vi "Tank1 GO!.vi"() -> ()   [LabVIEW 2012]
doc: "This VI demonstrates how to control a simulated Robotics Starter Kit 2.0 robot. With a few modifications, you can deploy this VI to the Single-Board RIO 9632 on a real robot, and it runs on the real-time controller. For more information about how to modify this VI so you can deploy it to real hardware, refer to the <B>Robotics Module>>Simulating Mobile Robots</B> book on the <B>Contents</B> tab of the LabVIEW Help."
uses:
  <vilib>/Platform/TimedLoop/XDataNode/timing_clust.ctl
  <vilib>/Platform/TimedLoop/XDataNode/nitl_modes.ctl
  <vilib>/Platform/TimedLoop/XDataNode/wakeup.ctl
  <vilib>/robotics/Starter Kit/2.0/9632 Host Interface/NI_Robotics_Starter Kit Host_9632_2.0.lvclass
  <vilib>/Utility/AngleManip/Degrees to Radians (Scalar DBL).vi
  <vilib>/FPGAPlugInAG/sbRIO-9632/niLvFpga_Open_sbRIO-9632.vi
  <vilib>/rvi/interface/common/dynamic/niFpgaDynamicAddResources.vi
  <vilib>/robotics/Steering/Steering Frame/Apply Steering Frame Velocity to Motors.vi
  <vilib>/FPGAPlugInAG/Dynamic/niLvFpga_Close_Dynamic.vi
  <vilib>/Platform/TimedLoop/XDataNode/XDataNode.xnode
  <vilib>/rvi/interface/nirviOpenFPGA/nirviOpenFPGA.xnode
  FPGA Bitfiles/mainframe_FPGATarget_FPGA-conrolofTan_P2Uk2TjUNj0.lvbitx
  <vilib>/rvi/interface/nirviCloseFPGA/nirviCloseFPGA.xnode
  <vilib>/Platform/TimedLoop/XDataNode/XDNodeRunTimeDep.lvlib
  <vilib>/Utility/AngleManip/NI_AngleManipulation.lvlib
  <vilib>/robotics/Utilities/Scan Angles/NI_Robotics_Scan Angles.lvlib
  <vilib>/robotics/Steering/Steering Frame/NI_Robotics_Steering Frame.lvclass
  <vilib>/robotics/Starter Kit/Host Interface/NI_Robotics_Starter Kit Host.lvclass
  <vilib>/robotics/Starter Kit/2.0/NI_Robotics_Starter Kit Host_2.0.lvlib
panel:
  out "Sensor Data":cluster{"angles (deg)":dbl[], "distances":dbl[]}(graph)
  in  "stop":bool
  # "This VI demonstrates how to control a simulated Robotics Starter Kit 2.0 robot.\n\nRun this VI to launch the simulation.  The simulated environment is displayed in a separate window.  The graph displays the range data acquired by the simulated ultrasonic sensor on the robot.  Click the STOP button to end the simulation."
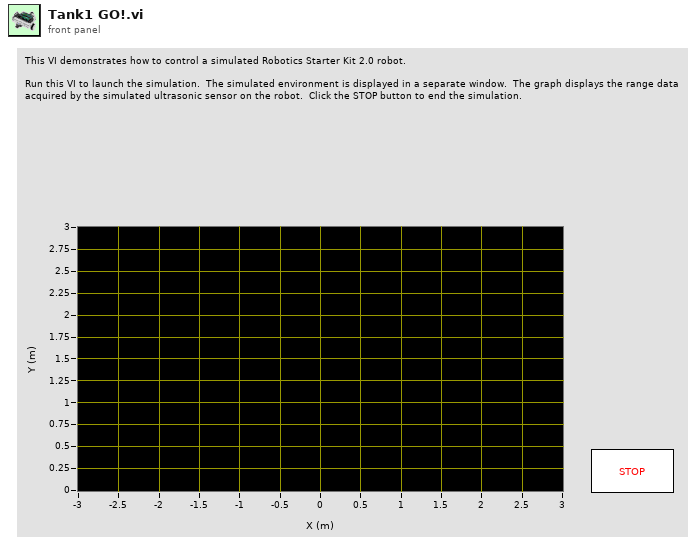
[diagram p1: front panel]
types:
  T1 = typedef "NI_Robotics_Scan Angles.lvlib/Scan Angle Data.ctl" = cluster{"angles":dbl[], "distances":dbl[], "current index":i32, "previous index":i32}
  T2 = typedef "XDNodeRunTimeDep.lvlib/timing_clust.ctl" = cluster{"Expected End [f-1]":u64, "Actual End [f-1]":u64, "Finished Late? [f-1]":bool, "Expected End [i-1]":u64, "Actual End [i-1]":u64, "Finished Late? [i-1]":bool, "Expected Start [i]":u64, "Actual Start [i]":u64, "Expected Start [f]":u64, "Actual Start [f]":u64, "Source Name":string, "Structure Name":string, "Period":i64, "Deadline":i64, "Offset":i64, "Start":i64, "Priority":i32, "Timeout":i32, "Mode":T3, "Wakeup Reason":T4, "Error":errorcluster, "Source Type":string, "Secondary Source Type":string, "Global End Time":u64, "Global Start Time":u64, "Frame Duration":u64, "Iteration Duration":u64, "Assigned CPU":i32, "I/O Scan Engine Mode":u32}
  T3 = typedef "XDNodeRunTimeDep.lvlib/nitl_modes.ctl" = enum32{"No Change", "Process missed periods, maintain original phase", "Discard missed periods, maintain original phase", "Process missed periods, ignore original phase", "Discard missed periods, ignore original phase"}
  T4 = typedef "XDNodeRunTimeDep.lvlib/wakeup.ctl" = enum32{"Normal", "Aborted", "Asynchronous wakeup", "Timing source error", "Timed loop error", "Timeout"}
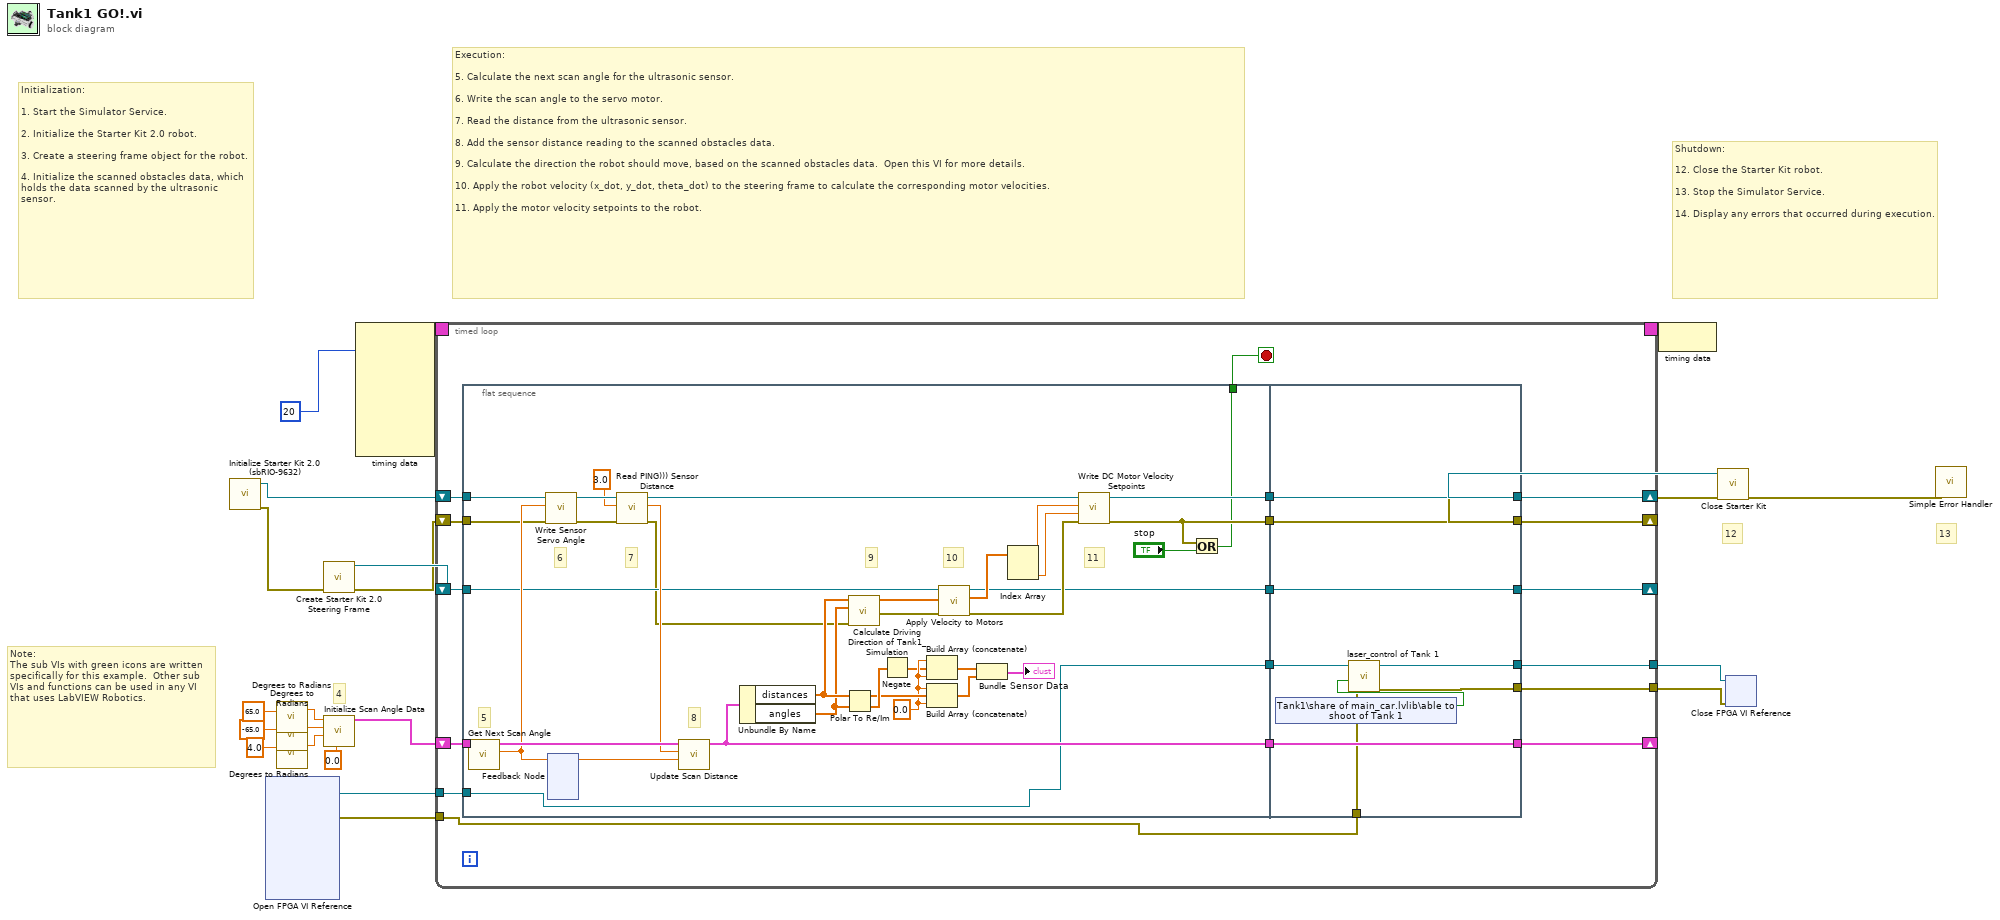
[diagram p0: block diagram]
diagram:
  # "13"
  # "12"
  # "Execution:\n\n5. Calculate the next scan angle for the ultrasonic sensor.\n\n6. Write the scan angle to the servo motor.\n\n7. Read the distance from the ultrasonic sensor.\n\n8. Add the sensor distance reading to the scanned obstacles data.\n\n9. Calculate the direction the robot should move, based on the scanned obstacles data.  Open this VI for more details.\n\n10. Apply the robot velocity (x_dot, y_dot, theta_dot) to the steering frame to calculate the corresponding motor velocities.\n\n11. Apply the motor velocity setpoints to the robot."
  # "Shutdown:\n\n12. Close the Starter Kit robot.\n\n13. Stop the Simulator Service.\n\n14. Display any errors that occurred during execution."
  # "Note:\nThe sub VIs with green icons are written specifically for this example.  Other sub VIs and functions can be used in any VI that uses LabVIEW Robotics."
  # "4"
  # "Initialization:\n\n1. Start the Simulator Service.\n\n2. Initialize the Starter Kit 2.0 robot.\n\n3. Create a steering frame object for the robot.\n\n4. Initialize the scanned obstacles data, which holds the data scanned by the ultrasonic sensor."
  n1 = call <vilib>:"Initialize Starter Kit 2.0 (sbRIO-9632).vi"() -> ("error out"=w6:errorcluster, "FPGA starter kit host 2.0 out"=w7:refnum<class "NI_Robotics_Starter Kit Host_9632_2.0.lvclass">)  [unwired: 10 in]
  n2 = xnode "Open FPGA VI Reference"() -> ("FPGA VI Reference Out"=w4:refnum<k20>, "error out"=w3:errorcluster)  [unwired: 2 in]
  n3 = call-poly <vilib>:"Degrees to Radians.vi"("angle (deg)"=65.0 ("max angle")) -> ("angle (rad)"=w15:dbl)  [unwired: 2 in]
  n4 = call-poly <vilib>:"Degrees to Radians.vi"("angle (deg)"=-65.0 ("min angle")) -> ("angle (rad)"=w11:dbl)  [unwired: 2 in]
  n5 = call-poly <vilib>:"Degrees to Radians.vi"("angle (deg)"=4.0 ("scan angle")) -> ("angle (rad)"=w12:dbl)  [unwired: 2 in]
  n6 = call <vilib>:"Create Starter Kit 2.0 Steering Frame.vi"("error in (no error)"=w6) -> ("error out"=w9:errorcluster, "starter kit differential steering frame"=w19:refnum<class "NI_Robotics_Differential Steering Frame.lvclass">)  [unwired: 9 in]
  n7 = call <vilib>:"Initialize Scan Angle Data.vi"("initial angle (0)"=0.0, "scan angle"=w12, "min angle"=w11, "max angle"=w15) -> ("scan angles"=w10:T1)  [unwired: 6 in, 1 out]
  n8 = node-c288(i64 20 ("Period")) -> (w22:T2)  [unwired: 6 in]
  n9 = timed-loop {
    shift-right: [w35] -> w18
    shift-left: w7 -> [w39]
    shift-right: [w33] -> w17
    shift-left: w9 -> [w36]
    shift-right: [w37] -> _
    shift-left: w19 -> [w38]
    timing: w22 -> [_]
    timing-out: [_] -> w21
    shift-right: [w34] -> _
    shift-left: w10 -> [w40]
    tunnel: w4 -> [w26]
    tunnel: w3 -> [w25]
    tunnel: [w24] -> w2
    tunnel: [w23] -> w1
    stop <- w32 stop-if-true
    n10 = flat-sequence {
      tunnel: w40 -> [w62]
      tunnel: w39 -> [w61]
      tunnel: w38 -> [w60]
      tunnel: w36 -> [w58]
      tunnel: [w42] -> w32
      tunnel: [w59] -> w31
      tunnel: [w57] -> w30
      tunnel: [w56] -> w29
      tunnel: [w46] -> w28
      tunnel: [w41] -> w27
      tunnel: w26 -> [w41]
      tunnel: [w81] -> w33
      tunnel: [w82] -> w34
      tunnel: [w83] -> w35
      tunnel: [w84] -> w37
      tunnel: w31 -> [w84]
      tunnel: w30 -> [w83]
      tunnel: w29 -> [w82]
      tunnel: w28 -> [w81]
      tunnel: w27 -> [w79]
      tunnel: w25 -> [w78]
      tunnel: [w77] -> w24
      tunnel: [w76] -> w23
      frame #0 {
        w52 = 0.0 ("element")
        # "7"
        # "6"
        # "11"
        # "10"
        # "9"
        # "8"
        # "5"
        n11 = call <vilib>:"Get Next Scan Angle.vi"("scan angles in"=w62) -> ("new angle"=w71:dbl, "scan angles out"=w74:T1)  [unwired: 9 in]
        n12 = call <vilib>:"Write Sensor Servo Angle.vi"("error in (no error)"=w58, "ccw servo angle (rad)"=w71, "starter kit host in"=w61) -> ("error out"=w68:errorcluster, "starter kit host out"=w69:refnum<class "NI_Robotics_Starter Kit Host_9632_2.0.lvclass">)  [unwired: 7 in]
        n13 = feedback #1() -> (w73:dbl)  [unwired: 1 in]
        n14 = feedback-in #1(w71) -> ()
        n15 = call <vilib>:"Read PING))) Sensor Distance.vi"("error in (no error)"=w68, "default distance (NaN)"=3.0, "starter kit host in"=w69) -> ("error out"=w45:errorcluster, "distance (m)"=w70:dbl, "starter kit host out"=w67:refnum<class "NI_Robotics_Starter Kit Host_9632_2.0.lvclass">)  [unwired: 5 in, 1 out]
        n16 = call <vilib>:"Update Scan Distance.vi"("scan angle"=w73, "new scan distance"=w70, "scan angles in"=w74) -> ("scan angles out"=w56:T1)  [unwired: 8 in]
        n17 = Unbundle By Name(w56) -> ("distances"=w48:dbl[], "angles"=w47:dbl[])
        n18 = Polar To Re/Im(2:w47, 3:w48) -> (0:w55:dbl[], 1:w54:dbl[])
        n19 = call "Calculate Driving Direction of Tank1_Simulation.vi"("error in (no error)"=w45, "obstacle angles (rad)"=w47, "obstacle distances (m)"=w48) -> ("error out"=w44:errorcluster, "steering frame velocity"=w43:dbl[])  [unwired: 7 in]
        n20 = Negate(x=w55) -> (-x=w50:dbl[])
        n21 = Build Array (concatenate)(w52, w50, w52) -> (w51:dbl[])
        n22 = Build Array (concatenate)(w52, w54, w52) -> (w53:dbl[])
        n23 = call-poly <vilib>:"Apply Velocity to Motors.vi"("error in (no error)"=w44, "steering frame velocity"=w43, "steering frame in"=w60) -> ("error out"=w66:errorcluster, "ccw motor velocity setpoints"=w72:dbl[], "steering frame out"=w59:refnum<class "NI_Robotics_Differential Steering Frame.lvclass">)  [unwired: 4 in, 2 out]
        n24 = Bundle(w51, w53) -> (→"Sensor Data":cluster{dbl[], dbl[]})  [unwired: 1 in]
        n25 = Index Array(array=w72) -> (element #1=w65:dbl, element #2=w64:dbl)  [unwired: 2 in]
        n26 = call <vilib>:"Write DC Motor Velocity Setpoints.vi"("error in (no error)"=w66, "right motor ccw velocity (rad/s)"=w64, "left motor ccw velocity (rad/s)"=w65, "starter kit host in"=w67) -> ("error out"=w46:errorcluster, "starter kit host out"=w57:refnum<class "NI_Robotics_Starter Kit Host_9632_2.0.lvclass">)  [unwired: 6 in]
        n27 = Or(x=w46, y="stop") -> (x .or. y?=w42:bool)
      }
      frame #1 {
        n28 = shared-variable "Tank1\\share of main_car.lvlib\\able to shoot of Tank 1"() -> (w80:bool)  [unwired: 1 in, 1 out]
        n29 = call "laser_control of Tank 1.vi"("error out"=w78, "Boolean"=w80, "FPGA VI Reference Out"=w79) -> ("error out 2"=w76:errorcluster, "FPGA VI Reference Out 2"=w77:refnum<k20>)  [unwired: 3 in]
      }
    }
  }
  n30 = node-c288(w21) -> ()
  n31 = call-dynamic "Close Starter Kit.vi"("error in (no error)"=w17, "starter kit host in"=w18) -> ("error out"=w5:errorcluster)  [unwired: 9 in]
  n32 = xnode "Close FPGA VI Reference"("FPGA VI Reference In"=w2, "error in"=w1) -> ()  [unwired: 1 out]
  n33 = call <vilib>:"Simple Error Handler.vi"("error in (no error)"=w5) -> ()  [unwired: 4 in, 5 out]
